vi "Brake Light Controller.vi"   [LabVIEW 2015]
uses:
  <vilib>/Platform/TimedLoop/XDataNode/timing_clust.ctl
  <vilib>/Platform/TimedLoop/XDataNode/nitl_modes.ctl
  <vilib>/Platform/TimedLoop/XDataNode/wakeup.ctl
  <vilib>/FPGAPlugInAG/sbRIO-9626/niLvFpga_Open_sbRIO-9626.vi
  <vilib>/rvi/interface/common/dynamic/niFpgaDynamicAddResources.vi
  Global Data.vi
  <vilib>/Utility/error.llb/Error Cluster From Error Code.vi
  <vilib>/rvi/errors/niLvFpgaAdjustHostInterfaceError.vi
  <vilib>/FPGAPlugInAG/Dynamic/niLvFpga_Close_Dynamic.vi
  <vilib>/Platform/TimedLoop/XDataNode/XDataNode.xnode
  <vilib>/rvi/interface/nirviOpenFPGA/nirviOpenFPGA.xnode
  FPGA Bitfiles/Latest.lvbitx
  <vilib>/rvi/interface/nirviReadWriteControl/nirviReadWriteControl.xnode
  <vilib>/rvi/interface/nirviCloseFPGA/nirviCloseFPGA.xnode
  <vilib>/Platform/TimedLoop/XDataNode/XDNodeRunTimeDep.lvlib
  <vilib>/rvi/interface/Simulation/niFpgaSimulationCallBeginRW.vi
  NiFpgaLv.dll
types:
  T1 = typedef "XDNodeRunTimeDep.lvlib/timing_clust.ctl" = cluster{"Expected End [f-1]":u64, "Actual End [f-1]":u64, "Finished Late? [f-1]":bool, "Expected End [i-1]":u64, "Actual End [i-1]":u64, "Finished Late? [i-1]":bool, "Expected Start [i]":u64, "Actual Start [i]":u64, "Expected Start [f]":u64, "Actual Start [f]":u64, "Source Name":string, "Structure Name":string, "Period":i64, "Deadline":i64, "Offset":i64, "Start":i64, "Priority":i32, "Timeout":i32, "Mode":T2, "Wakeup Reason":T3, "Error":errorcluster, "Source Type":string, "Secondary Source Type":string, "Global End Time":u64, "Global Start Time":u64, "Frame Duration":u64, "Iteration Duration":u64, "Assigned CPU":i32, "I/O Scan Engine Mode":u32}
  T2 = typedef "XDNodeRunTimeDep.lvlib/nitl_modes.ctl" = enum32{"No Change", "Process missed periods, maintain original phase", "Discard missed periods, maintain original phase", "Process missed periods, ignore original phase", "Discard missed periods, ignore original phase"}
  T3 = typedef "XDNodeRunTimeDep.lvlib/wakeup.ctl" = enum32{"Normal", "Aborted", "Asynchronous wakeup", "Timing source error", "Timed loop error", "Timeout"}
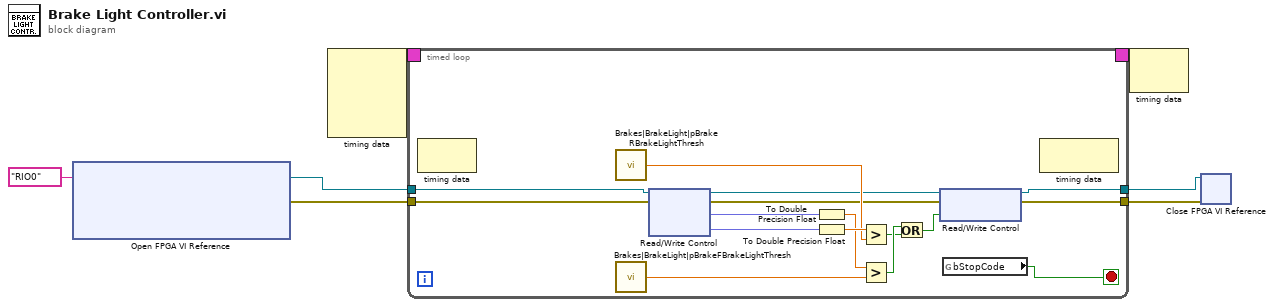
[diagram p0: block diagram]
diagram:
  n1 = xnode "Open FPGA VI Reference"("resource name"=tag "RIO0") -> ("FPGA VI Reference Out"=w5:refnum<k20>, "error out"=w4:errorcluster)  [unwired: 1 in]
  n2 = node-c288() -> (w7:T1)  [unwired: 4 in]
  n3 = timed-loop {
    timing: w7 -> [_]
    timing-out: [_] -> w6
    tunnel: w5 -> [w23]
    tunnel: w4 -> [w22]
    tunnel: [w10] -> w3
    tunnel: [w9] -> w2
    stop <- w8 stop-if-true
    n4 = node-c288() -> ()  [unwired: 1 in, 1 out]
    n5 = call "Brakes|BrakeLight|pBrakeRBrakeLightThresh"() -> ("Value"=w17:sgl)
    n6 = call "Brakes|BrakeLight|pBrakeFBrakeLightThresh"() -> ("Value"=w16:sgl)
    n7 = xnode "Read/Write Control"("FPGA VI Reference In"=w23, "error in"=w22) -> ("FPGA VI Reference Out"=w13:refnum<k20>, "error out"=w12:errorcluster, "pBrakeF"=w21:fxp<+,26,13>, "pBrakeR"=w20:fxp<+,26,13>)
    n8 = To Double Precision Float(number=w21) -> (double precision float=w18:dbl)
    n9 = To Double Precision Float(number=w20) -> (double precision float=w19:dbl)
    n10 = Greater?(x=w19, y=w17) -> (0:w14:bool)
    n11 = Greater?(x=w18, y=w16) -> (0:w15:bool)
    n12 = Or(x=w15, y=w14) -> (x .or. y?=w11:bool)
    n13 = xnode "Read/Write Control"("FPGA VI Reference In"=w13, "error in"=w12, "bBrakeLight"=w11) -> ("FPGA VI Reference Out"=w10:refnum<k20>, "error out"=w9:errorcluster)
    n14 = global read "Global Data.vi" "bStopCode"() -> (w8:bool)
    n15 = node-c288() -> ()  [unwired: 1 in, 1 out]
  }
  n16 = node-c288(w6) -> ()  [unwired: 1 out]
  n17 = xnode "Close FPGA VI Reference"("FPGA VI Reference In"=w3, "error in"=w2) -> ()  [unwired: 1 out]
